vi "TestControllerPC.vi"() -> ()   [LabVIEW 2010]
uses:
  <vilib>/picture/picture.llb/Draw True-Color Pixmap.vi
panel:
  in  "Select  a \"Controller\"":u16(ring) items=["Random", "Cosntant", "Multiply by 2", "Increase by 1"]
  in  "Should the Read block the model?":bool
  out "Counter Send/receive":dynamicdata(graph)
  out "bytes read":i32
  in  "Enable Read":bool=TRUE
  out "Packet Payload":string
  in  "Write packet":bool=TRUE
  in  "When do you want to send?":u16(ring) items=["Manually", "Automatically"]
  out "Bytes written":dbl format="%.2f"
  out "Packet Sent":string
  in  "Port Number":i32=9002
  out "KTH  Automatic Control \nTemplates. Test Controller in the PC":picture
  # "READ PACKET"
  # "For TestSerialCommMsg:\nheaderSize = 9\npayload = 4"
  # "CONTROLLER"
  # "It is not a controller, but it modifies the last received data and send the a new value.\nIt could be a template for a scenario where the controller needs to be implemented\non the PC"
  # "Communication control"
  # "WRITE PACKET"
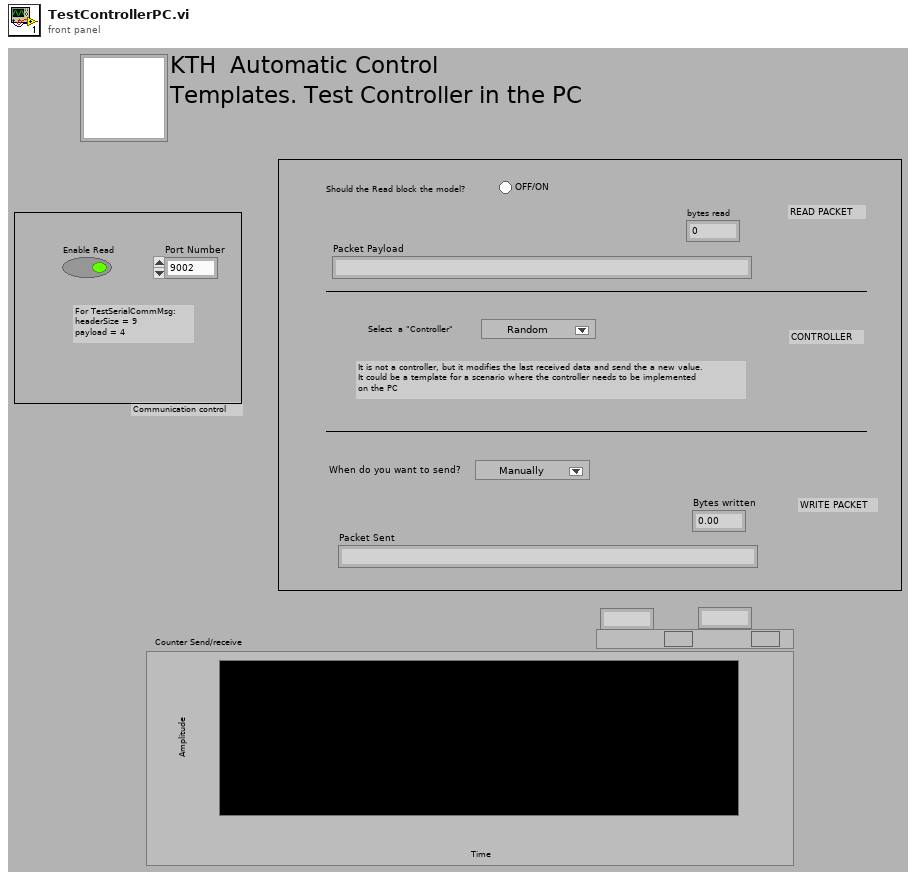
[diagram p1: front panel]
types:
  T1 = typedef "imagedata.ctl" = cluster{"image type":i32, "image depth":i32, "image":u8[], "mask":u8[], "colors":u32[], "Rectangle":cluster{"left":i16, "top":i16, "right":i16, "bottom":i16}}
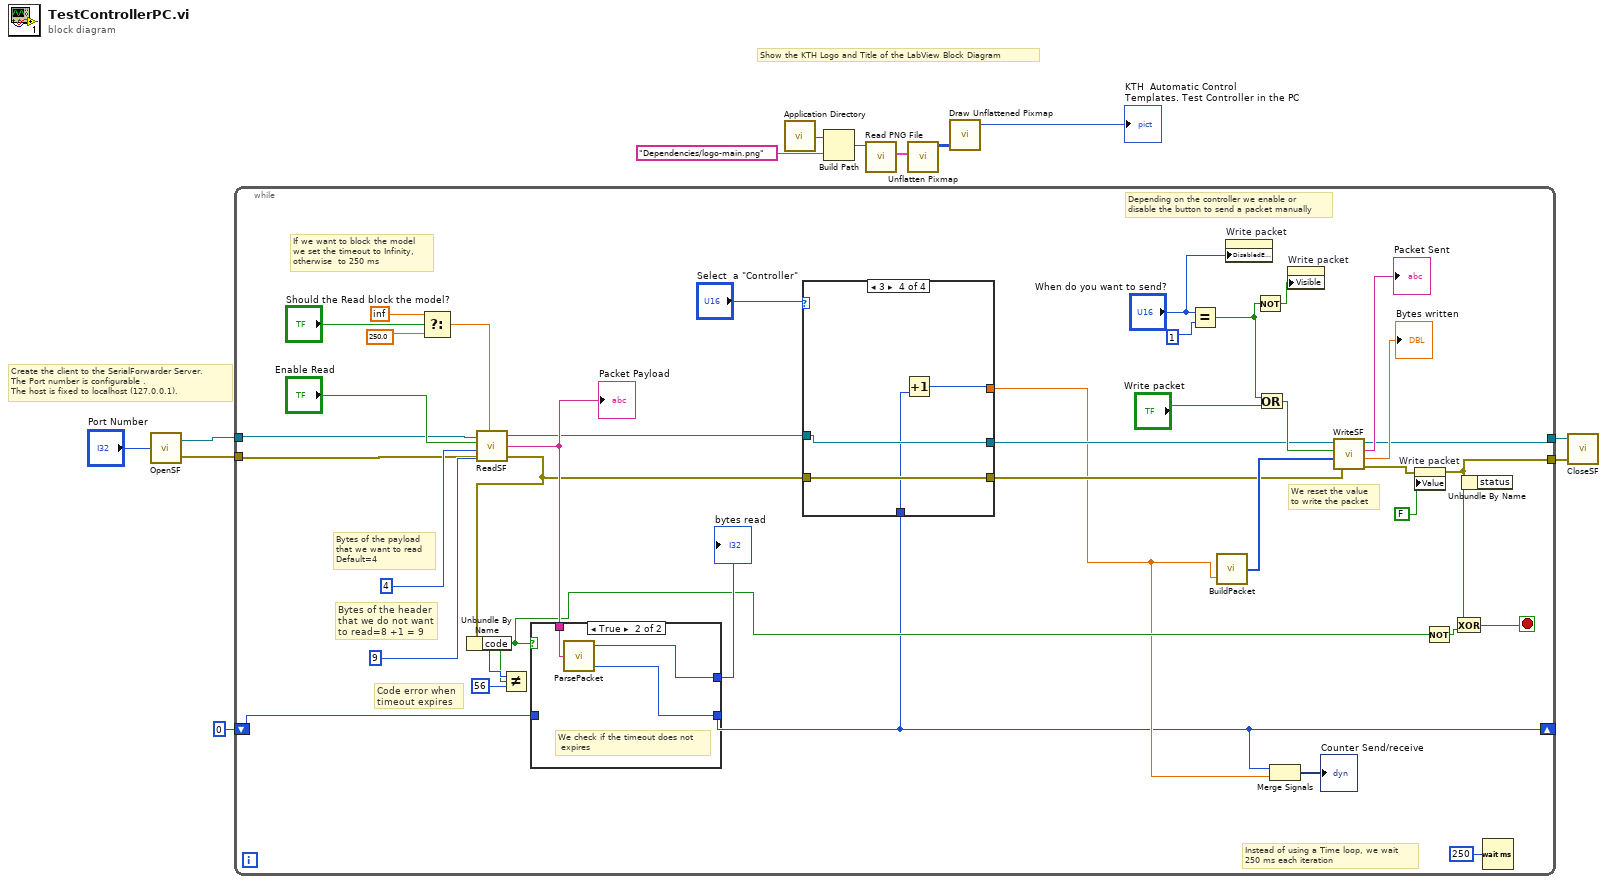
[diagram p0: block diagram]
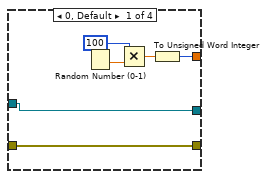
[diagram p2: hidden frame]
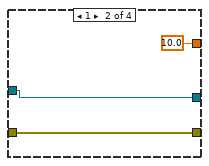
[diagram p3: hidden frame]
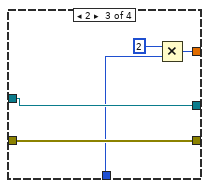
[diagram p4: hidden frame]
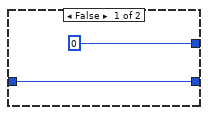
[diagram p5: hidden frame]
diagram:
  # "Create the client to the SerialForwarder Server.\nThe Port number is configurable . \nThe host is fixed to localhost (127.0.0.1)."
  # "Show the KTH Logo and Title of the LabView Block Diagram"
  n1 = call "OpenSF.vi"("Port Number"="Port Number") -> ("error out"=w11:errorcluster, "connection ID"=w12:refnum<k5>)
  n2 = while {
    tunnel: w12 -> [w28]
    tunnel: w11 -> [w27]
    tunnel: [w22] -> w10
    tunnel: [w21] -> w9
    shift-right: [w13] -> _
    shift-left: i16 0 ("Counter") -> [w14]
    stop <- w25 stop-if-true
    # "If we want to block the model\nwe set the timeout to Infinity, \notherwise  to 250 ms"
    # "Code error when  \ntimeout expires"
    # "Bytes of the payload \nthat we want to read\nDefault=4"
    # "Bytes of the header\nthat we do not want \nto read=8 +1 = 9"
    # "We reset the value\nto write the packet"
    # "Depending on the controller we enable or\ndisable the button to send a packet manually"
    # "Instead of using a Time loop, we wait \n250 ms each iteration"
    n3 = Select(t=inf, s="Should the Read block the model?", f=250.0 ("timeout (optional)")) -> (s? t:f=w29:dbl)
    n4 = call "ReadSF.vi"("connection ID in"=w28, "error in"=w27, "enabled"="Enable Read", "bytes to read"=4, "timeout (optional)"=w29, "header size"=9 ("bytes to read")) -> ("connection ID out"=w19:refnum<k5>, "string"=w39:string, "error out"=w18:errorcluster)
    "Packet Payload" <- w39
    n5 = Unbundle By Name(w18) -> ("code"=w35:i32)
    n6 = Not Equal?(x=w35, y=56) -> (x != y?=w24:bool)
    n7 = case shown="True" w24 {
      tunnel: w39 -> [_ w75]
      tunnel: [0 ("Bytes read") w74] -> w33
      tunnel: [w71 w73] -> w13
      tunnel: w14 -> [w71 _]
      frame False {
      }
      frame True {
        # "We check if the timeout does not\n expires"
        n8 = call "ParsePacket.vi"("data out"=w75) -> ("Counter"=w73:i16, "Bytes read"=w74:i32)  [unwired: 1 out]
      }
    }
    "bytes read" <- w33
    n9 = case shown="3" "Select  a \"Controller\"" {
      tunnel: w19 -> [w57 w60 w65 w69]
      tunnel: w18 -> [w58 w61 w66 w70]
      tunnel: [w58 w61 w66 w70] -> w17
      tunnel: [w57 w60 w65 w69] -> w16
      tunnel: [w54 10.0 w64 w68] -> w15
      tunnel: w13 -> [_ _ w63 w67]
      frame 0, Default {
        n10 = Random Number (0-1)() -> (number: 0 to 1=w56:dbl)
        n11 = Multiply(x=u16 100, y=w56) -> (x*y=w53:dbl)
        n12 = To Unsigned Word Integer(number=w53) -> (unsigned 16bit integer=w54:u16)
      }
      frame 1 {
      }
      frame 2 {
        n13 = Multiply(x=i16 2, y=w63) -> (x*y=w64:i16)
      }
      frame 3 {
        n14 = Increment(x=w67) -> (x+1=w68:i16)
      }
    }
    n15 = Equal?(x="When do you want to send?", y=u16 1) -> (x = y?=w41:bool)
    n16 = call "BuildPacket.vi"("Counter"=w15) -> ("PacketArray"=w52:i32[])  [unwired: 1 in]
    n17 = property on="Write packet" class="Bool (strict)"("DisabledEnum"="When do you want to send?") -> ()  [unwired: 2 in, 2 out]
    n18 = Not(x=w41) -> (.not. x?=w42:bool)
    n19 = Or(x=w41, y="Write packet") -> (x .or. y?=w47:bool)
    n20 = Merge Signals(w13, w15) -> (→"Counter Send/receive":dynamicdata)
    n21 = property on="Write packet" class="Bool (strict)"("Visible"=w42) -> ()  [unwired: 2 in, 2 out]
    n22 = call "WriteSF.vi"("error in"=w17, "packet"=w52, "Enablle write"=w47, "connection ID"=w16) -> ("error out"=w45:errorcluster, "Bytes written to SF"=→"Bytes written":dbl, "Packet String"=→"Packet Sent":string, "connection ID out"=w22:refnum<k5>)
    n23 = property on="Write packet" class="Bool (strict)"(error in=w45, "Value"=FALSE ("Write packet")) -> (error out=w21:errorcluster)  [unwired: 1 in, 1 out]
    n24 = Not(x=w24) -> (.not. x?=w26:bool)
    n25 = Unbundle By Name(w21) -> ("status"=w23:bool)
    n26 = Exclusive Or(1:w26, 2:w23) -> (0:w25:bool)
    n27 = Wait (ms)(milliseconds to wait=u32 250) -> ()  [unwired: 1 out]
  }
  n28 = call <vilib>:"Application Directory.vi"() -> ("Application Directory"=w4:path)
  n29 = Build Path(base path=w4, name or relative path="Dependencies/logo-main.png") -> (appended path=w5:path)
  n30 = call <vilib>:"Read PNG File.vi"("path to PNG file"=w5) -> ("image data"=w8:T1)  [unwired: 8 in, 2 out]
  n31 = call <vilib>:"Unflatten Pixmap.vi"("image data"=w8) -> ("24-bit pixmap"=w7:u32[][])  [unwired: 4 in, 6 out]
  n32 = call-poly <vilib>:"Draw Unflattened Pixmap.vi"("data (RGB format)"=w7) -> ("new picture"=→"KTH  Automatic Control \nTemplates. Test Controller in the PC":picture)  [unwired: 8 in]
  n33 = call "CloseSF.vi"("error out"=w9, "connection ID"=w10) -> ()  [unwired: 1 in]
